vi "Get Result Code.vi"(5 "Headers":string, 11 "error in (no error)":errorcluster) -> (6 "Status Code":i32, 15 "error out":errorcluster)   [LabVIEW 2016]
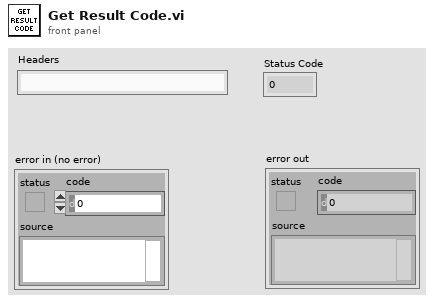
[diagram p1: front panel]
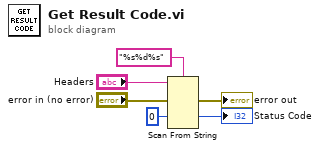
[diagram p0: block diagram]
diagram:
  n1 = Scan From String(format string="%s%d%s", input string="Headers", error in="error in (no error)", default 2=0 ("default value 2")) -> (error out=→"error out":errorcluster, output 2=→"Status Code":i32)  [unwired: 5 in, 2 out]
